vi "LED_test1.vi"() -> ()   [LabVIEW 2012]
uses:
  <vilib>/Utility/file.llb/Read From Spreadsheet File (DBL).vi
  <vilib>/gmath/NI_Gmath.lvlib
  <vilib>/Analysis/NI_AALPro.lvlib
panel:
  out "x2":dbl=3e-06
  out "x1":dbl=3e-06
  out "WL_1":dbl
  out "WL_2":dbl
  in  "WL2":dbl
  in  "WL1":dbl
  out "EQE_array":dbl[](array[numeric])
  out "XY Graph 4":T1(graph)
  out "XY Graph 3":cluster{"Wavelength":dbl[], "Counts":dbl[]}(graph)
  out "Luminance Ratio":dbl[](array[numeric])
  out "Calculated_luminance_array":dbl[](array[numeric])
  out "Calculated_candela_array":dbl[](array[numeric])
  out "Photon_count_array":dbl[](array[numeric])
  out "Photon_count":dbl
  out "Energy_WL":dbl[](array[numeric])
  out "Calculated_candela":dbl
  out "Abs_irr_itpl":dbl[](array[numeric]) format="%_6g"
  out "WL itpl 2":dbl[](array[numeric]) format="%_6g"
  out "Luminous Power Efficiency":dbl[](array[numeric])
  out "current efficiency (Cd/A)":dbl[](array[numeric])
  out "current density (mA/cm2)":dbl[](array[numeric])
  in  "Device Area (m2)":dbl=3e-06
  out "WL_spectrum":dbl[](array[numeric])
  out "Counts_spectrum":dbl[](array[numeric])
  out "Abs_Irr_spectrum":dbl[](array[numeric])
  out "subarray 2":dbl[][](array[numeric])
  out "Counts_dark_spectrum":dbl[](array[numeric])
  out "WL_dark_spectrum":dbl[](array[numeric])
  out "Dark Spectrum all":dbl[][](array[numeric]) format="%0.3f"
  out "Dark_spectrum":dbl[][](array[numeric])
  out "All Spectrum":dbl[][](array[numeric])
  in  "Spectrum File":path=path "W:/LED_quickVIEW/For calibration/20170914_194634spectrum_raw.ciemo"
  out "uW":dbl[](array[numeric])
  out "Luminance":dbl[](array[numeric])
  out "Candela":dbl[](array[numeric])
  out "Current":dbl[](array[numeric])
  out "Voltage":dbl[](array[numeric])
  out "Data":dbl[][](array[numeric]) format="%#.3e"
  out "Waveform Graph":T2(graph)
  in  "Data File":path=path "W:/LED_quickVIEW/For calibration/20170914_194634data.ciemo"
  in  "Calibration File":path=path "W:/LED_quickVIEW/For calibration/2016-12-19 callibration_OOIIrrad.cal_OOIIrrad.cal_OOIIrrad.cal"
  in  "Dark Spectrum File":path=path "W:/LED_quickVIEW/For calibration/20170914_194634dark_reference.ciemo"
  out "max value":dbl
  out "Peak Position":dbl
  out "max index(es)":i32
  out "Iso. Coef. itpl":dbl[](array[numeric]) format="%_6g"
  out "WL itpl":dbl[](array[numeric]) format="%_6g"
  out "XY Graph 2":cluster{"WL":dbl[], "Iso. Coef.":dbl[]}[](graph)
  out "Iso. Coef.":dbl[](array[numeric])
  out "WL":dbl[](array[numeric])
  out "Wavelength":dbl[](array[numeric])
  out "Counts to Abs Irr":dbl[](array[numeric])
  out "XY Graph":cluster{"Wavelength":dbl[], "Counts":dbl[]}(graph)
  out "subarray":dbl[][](array[numeric])
  out "array":dbl[][](array[numeric])
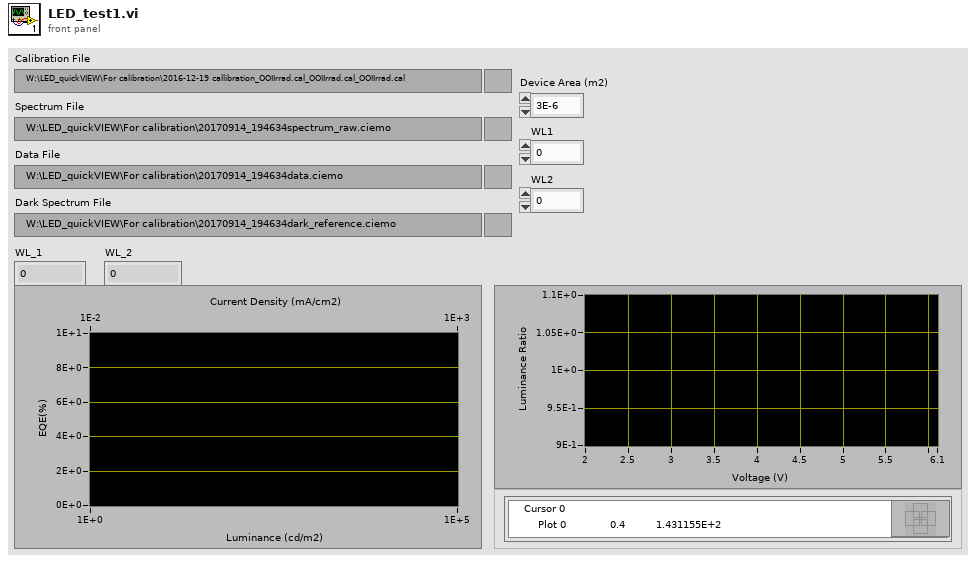
[diagram p1: front panel]
types:
  T1 = cluster{"current density (mA/cm2)":dbl[], "EQE_array":dbl[]}[]
  T2 = cluster{"min value":dbl, "min value":dbl, "Iso. Coef. itpl":dbl[]}
  T3 = cluster{"Wavelength":dbl[], "Counts to Abs Irr":dbl[]}
  T4 = cluster{"WL itpl":dbl[], "Iso. Coef. itpl":dbl[]}
  T5 = cluster{"WL itpl":dbl[], "Iso. Coef. itpl":dbl[]}[]
  T6 = cluster{"current density (mA/cm2)":dbl[], "EQE_array":dbl[]}
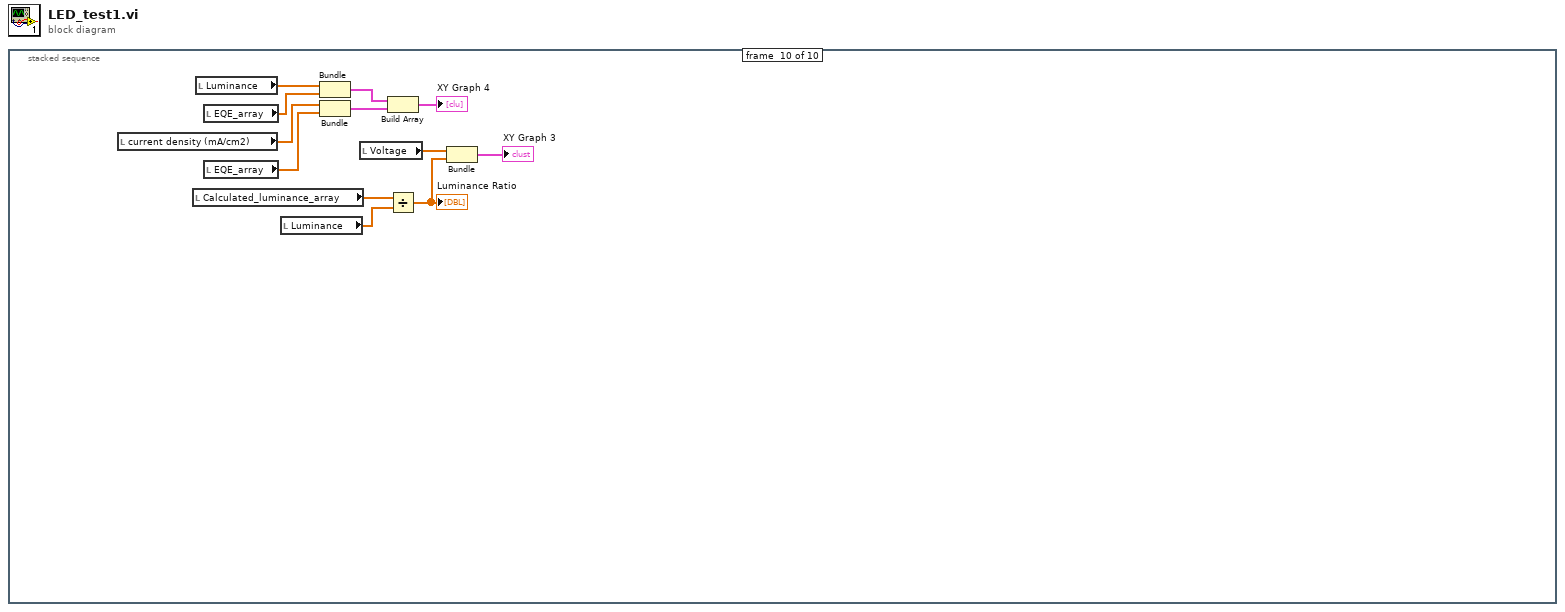
[diagram p0: block diagram]
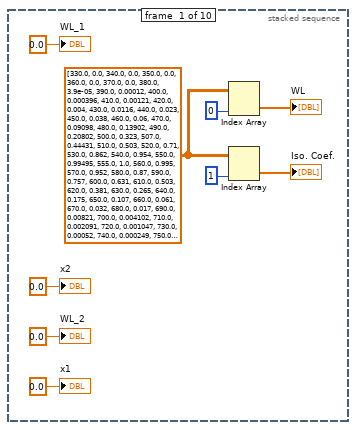
[diagram p2: hidden frame]
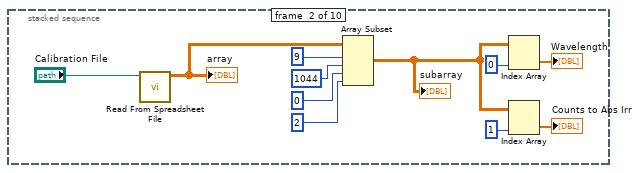
[diagram p3: hidden frame]
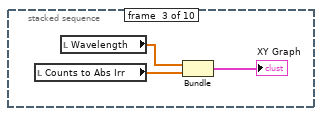
[diagram p4: hidden frame]
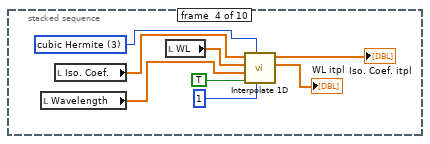
[diagram p5: hidden frame]
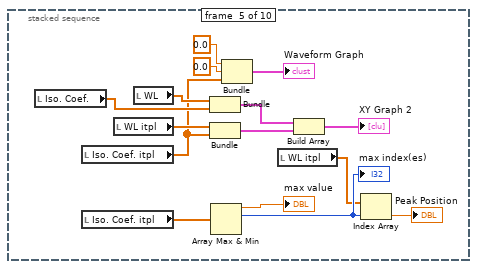
[diagram p6: hidden frame]
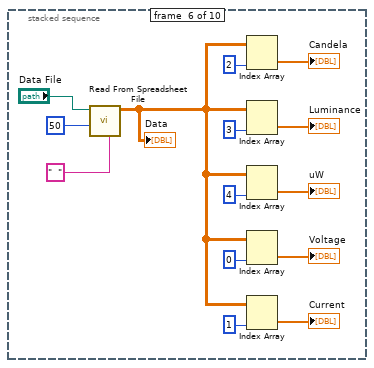
[diagram p7: hidden frame]
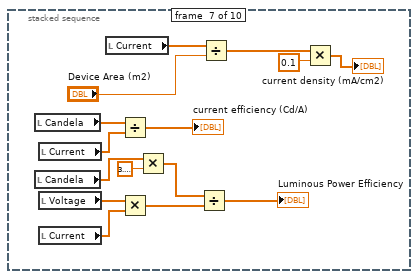
[diagram p8: hidden frame]
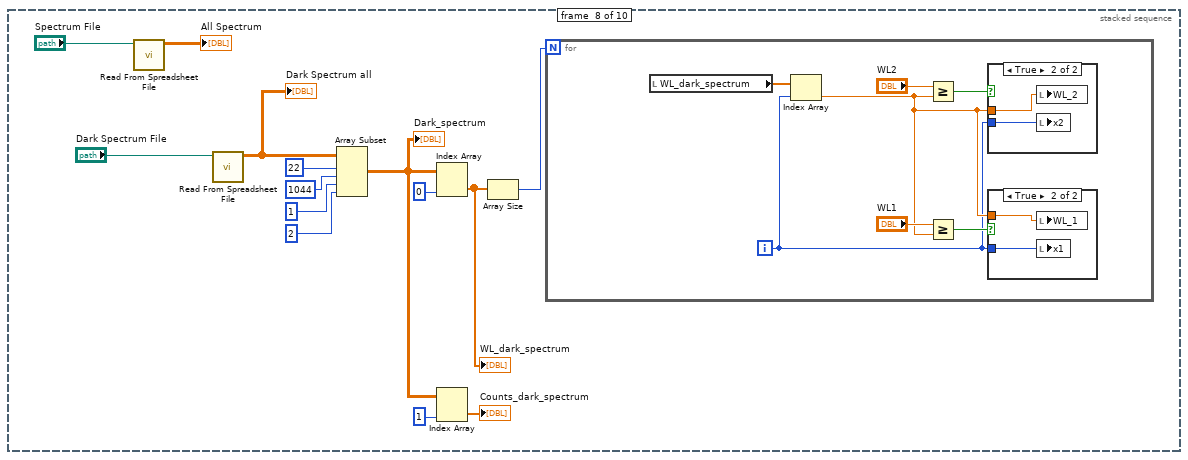
[diagram p9: hidden frame]
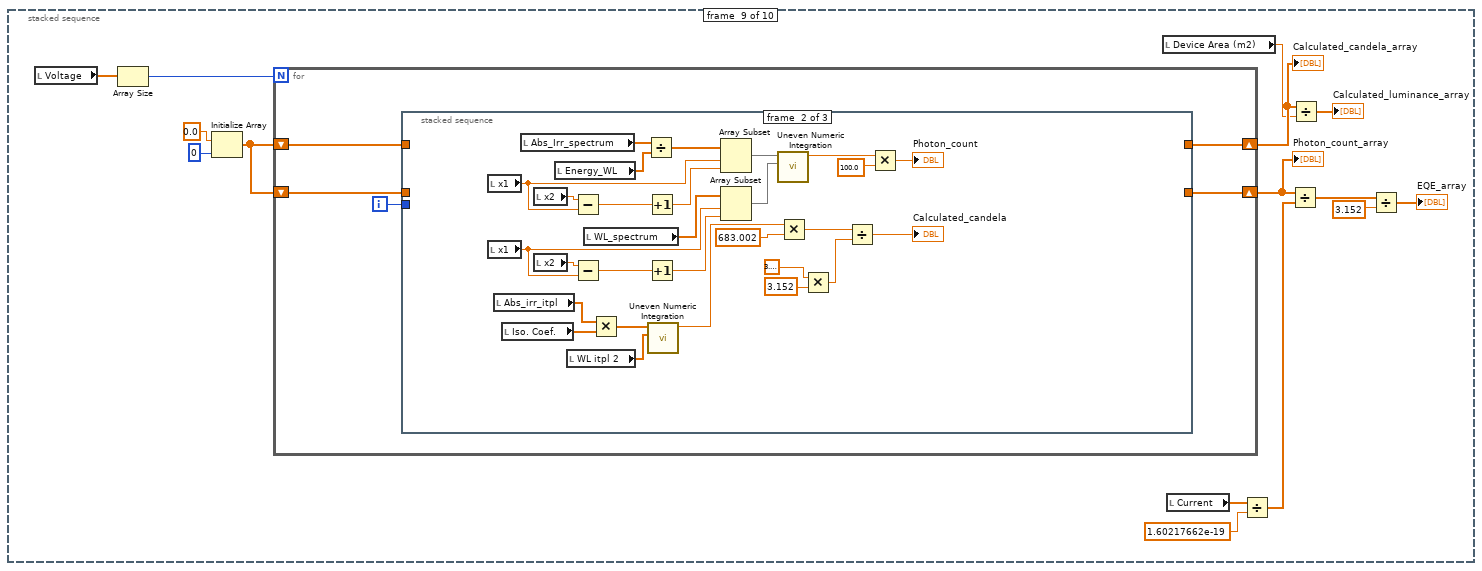
[diagram p12: hidden frame]
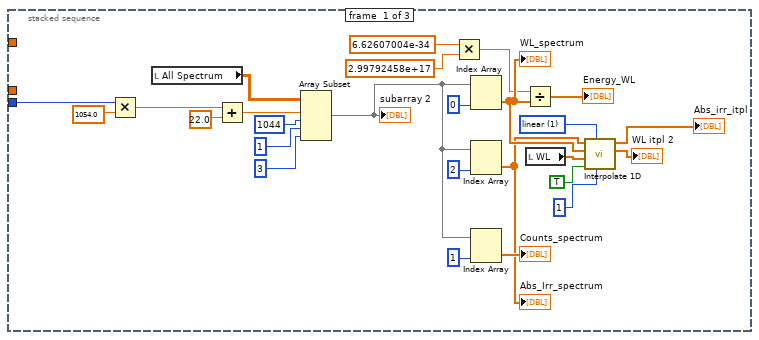
[diagram p13: hidden frame]
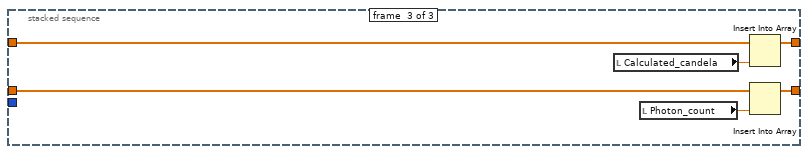
[diagram p14: hidden frame]
diagram:
  n1 = stacked-sequence {
    frame #0 {
      w8 = dbl[][] [[330.0, 0.0], [340.0, 0.0], [350.0, 0.0], [360.0, 0.0], [370.0, 0.0], [380.0, 3.9e-05], [390.0, 0.00012], [400.0, 0.000396], [410.0, 0.00121], [420.0, 0.004], [430.0, 0.0116], [440.0, 0.023], [450.0, 0.038], [460.0, 0.06], [470.0, 0.09098], [480.0, 0.13902], [490.0, 0.20802], [500.0, 0.323], [507.0, 0.44431], [510.0, 0.503], [520.0, 0.71], [530.0, 0.862], [540.0, 0.954], [550.0, 0.99495], [555.0, 1.0], [560.0, 0.995], [570.0, 0.952], [580.0, 0.87], [590.0, 0.757], [600.0, 0.631], [610.0, 0.503], [620.0, 0.381], [630.0, 0.265], [640.0, 0.175], [650.0, 0.107], [660.0, 0.061], [670.0, 0.032], [680.0, 0.017], [690.0, 0.00821], [700.0, 0.004102], [710.0, 0.002091], [720.0, 0.001047], [730.0, 0.00052], [740.0, 0.000249], [750.0, 0.00012], [760.0, 6e-05], [770.0, 3e-05], [780.0, 0.0], [790.0, 0.0], [800.0, 0.0], [810.0, 0.0], [820.0, 0.0], [830.0, 0.0], [840.0, 0.0], [850.0, 0.0], [860.0, 0.0], [870.0, 0.0], [880.0, 0.0], [890.0, 0.0], [900.0, 0.0], [910.0, 0.0], [920.0, 0.0], [930.0, 0.0], [940.0, 0.0], [950.0, 0.0], [960.0, 0.0], [970.0, 0.0], [980.0, 0.0], [990.0, 0.0], [1000.0, 0.0], [1010.0, 0.0], [1020.0, 0.0], [1030.0, 0.0], [1040.0, 0.0], [1050.0, 0.0], [1060.0, 0.0], [1070.0, 0.0], [1080.0, 0.0], [1090.0, 0.0], [1100.0, 0.0], [1110.0, 0.0], [1120.0, 0.0], [1130.0, 0.0], [1140.0, 0.0]] ("all rows")
      n2 = Index Array(array=w8, index (col)=0 ("disabled index (col)")) -> (element=→"WL":dbl[])  [unwired: 1 in]
      n3 = Index Array(array=w8, index (col)=1 ("disabled index (col)")) -> (element=→"Iso. Coef.":dbl[])  [unwired: 1 in]
      "WL_2" <- 0.0 ("WL_2")
      "WL_1" <- 0.0 ("WL_1")
      "x1" <- 0.0 ("x1")
      "x2" <- 0.0 ("x2")
    }
    frame #1 {
      n4 = call-poly <vilib>:"Read From Spreadsheet File.vi"("file path (dialog if empty)"="Calibration File") -> ("all rows"=w17:dbl[][])  [unwired: 6 in, 4 out]
      "array" <- w17
      n5 = Array Subset(array=w17, index (row)=9 ("index"), length (row)=1044 ("length"), index (col)=0 ("index"), length (col)=2 ("length")) -> (w14:dbl[][])
      "subarray" <- w14
      n6 = Index Array(array=w14, index (col)=0 ("index")) -> (element=→"Wavelength":dbl[])  [unwired: 1 in]
      n7 = Index Array(array=w14, index (col)=1 ("length")) -> (element=→"Counts to Abs Irr":dbl[])  [unwired: 1 in]
    }
    frame #2 {
      n8 = local read "Counts to Abs Irr"() -> (w21:dbl[])
      n9 = local read "Wavelength"() -> (w22:dbl[])
      n10 = Bundle("Wavelength"=w22, "Counts to Abs Irr"=w21) -> (→"XY Graph":T3)  [unwired: 1 in]
    }
    frame #3 {
      w27 = 3 items=["nearest", "linear", "spline", "cubic Hermite", "Lagrange"] ("method")
      n11 = local read "Wavelength"() -> (w29:dbl[])
      n12 = local read "Iso. Coef."() -> (w30:dbl[])
      n13 = local read "WL"() -> (w31:dbl[])
      n14 = call <vilib>:"Interpolate 1D.vi"("ntimes"=1, "method"=w27, "X is monotonic"=TRUE, "xi"=w29, "X"=w31, "Y"=w30) -> ("xi used"=→"WL itpl":dbl[], "yi"=→"Iso. Coef. itpl":dbl[])  [unwired: 3 in, 1 out]
    }
    frame #4 {
      n15 = local read "Iso. Coef."() -> (w46:dbl[])
      n16 = local read "Iso. Coef. itpl"() -> (w34:dbl[])
      n17 = local read "Iso. Coef. itpl"() -> (w39:dbl[])
      n18 = local read "WL itpl"() -> (w43:dbl[])
      n19 = local read "WL"() -> (w45:dbl[])
      n20 = Bundle("WL"=w45, "Iso. Coef."=w46) -> (w44:cluster{"WL":dbl[], "Iso. Coef.":dbl[]})  [unwired: 1 in]
      n21 = Bundle("WL itpl"=w43, "Iso. Coef. itpl"=w34) -> (w36:T4)  [unwired: 1 in]
      n22 = Array Max & Min(array=w39) -> (max value=→"max value":dbl, max index (indices)=w42:i32)  [unwired: 2 out]
      "max index(es)" <- w42
      n23 = Bundle("min value"=0.0, "min value"=0.0, "Iso. Coef. itpl"=w34) -> (→"Waveform Graph":T2)  [unwired: 1 in]
      n24 = local read "WL itpl"() -> (w41:dbl[])
      n25 = Build Array(w44, w36) -> (→"XY Graph 2":T5)
      n26 = Index Array(array=w41, index=w42) -> (element=→"Peak Position":dbl)
    }
    frame #5 {
      n27 = call-poly <vilib>:"Read From Spreadsheet File.vi"("delimiter (\\t)"="  " ("delimiter (\\t)"), "start of read offset (chars.:0)"=50, "file path (dialog if empty)"="Data File") -> ("all rows"=w47:dbl[][])  [unwired: 4 in, 4 out]
      "Data" <- w47
      n28 = Index Array(array=w47, index (col)=2 ("index (row)")) -> (element=→"Candela":dbl[])  [unwired: 1 in]
      n29 = Index Array(array=w47, index (col)=3 ("index (row)")) -> (element=→"Luminance":dbl[])  [unwired: 1 in]
      n30 = Index Array(array=w47, index (col)=4 ("index (row)")) -> (element=→"uW":dbl[])  [unwired: 1 in]
      n31 = Index Array(array=w47, index (col)=0 ("index (row)")) -> (element=→"Voltage":dbl[])  [unwired: 1 in]
      n32 = Index Array(array=w47, index (col)=1 ("index (row)")) -> (element=→"Current":dbl[])  [unwired: 1 in]
    }
    frame #6 {
      n33 = local read "Candela"() -> (w70:dbl[])
      n34 = local read "Candela"() -> (w63:dbl[])
      n35 = local read "Current"() -> (w71:dbl[])
      n36 = local read "Voltage"() -> (w65:dbl[])
      n37 = local read "Current"() -> (w64:dbl[])
      n38 = local read "Current"() -> (w68:dbl[])
      n39 = Divide(x=w70, y=w71) -> (x/y=→"current efficiency (Cd/A)":dbl[])
      n40 = Multiply(x=w65, y=w64) -> (x*y=w67:dbl[])
      n41 = Multiply(x=w63, y=3.141592653589793) -> (x*y=w66:dbl[])
      n42 = Divide(x=w66, y=w67) -> (x/y=→"Luminous Power Efficiency":dbl[])
      n43 = Divide(x=w68, y="Device Area (m2)") -> (x/y=w73:dbl[])
      n44 = Multiply(x=w73, y=0.1) -> (x*y=→"current density (mA/cm2)":dbl[])
    }
    frame #7 {
      n45 = call-poly <vilib>:"Read From Spreadsheet File.vi"("file path (dialog if empty)"="Spectrum File") -> ("all rows"=→"All Spectrum":dbl[][])  [unwired: 6 in, 4 out]
      n46 = call-poly <vilib>:"Read From Spreadsheet File.vi"("file path (dialog if empty)"="Dark Spectrum File") -> ("all rows"=w86:dbl[][])  [unwired: 6 in, 4 out]
      "Dark Spectrum all" <- w86
      n47 = Array Subset(array=w86, index (row)=22 ("index"), length (row)=1044 ("length"), index (col)=1 ("index"), length (col)=2 ("length")) -> (w78:dbl[][])
      "Dark_spectrum" <- w78
      n48 = Index Array(array=w78, index (col)=0 ("index")) -> (element=w77:dbl[])  [unwired: 1 in]
      "WL_dark_spectrum" <- w77
      n49 = Index Array(array=w78, index (col)=1 ("index")) -> (element=→"Counts_dark_spectrum":dbl[])  [unwired: 1 in]
      n50 = Array Size(array=w77) -> (size(s)=w76:i32)
      n51 = for {
        N: w76 -> [_]
        i -> [w90]
        n52 = local read "WL_dark_spectrum"() -> (w92:dbl[])
        n53 = Index Array(array=w92, index=w90) -> (element=w91:dbl)
        n54 = Greater Or Equal?(x="WL2", y=w91) -> (x >= y?=w94:bool)
        n55 = Greater Or Equal?(x="WL1", y=w91) -> (x >= y?=w93:bool)
        n56 = case shown="True" w94 {
          tunnel: w91 -> [_ w100]
          tunnel: w90 -> [_ w99]
          frame False {
          }
          frame True {
            n57 = local write "WL_2"(w100) -> ()
            n58 = local write "x2"(w99) -> ()
          }
        }
        n59 = case shown="True" w93 {
          tunnel: w91 -> [_ w98]
          tunnel: w90 -> [_ w97]
          frame False {
          }
          frame True {
            n60 = local write "WL_1"(w98) -> ()
            n61 = local write "x1"(w97) -> ()
          }
        }
      }
    }
    frame #8 {
      n62 = local read "Voltage"() -> (w115:dbl[])
      n63 = Array Size(array=w115) -> (size(s)=w114:i32)
      n64 = Initialize Array(0.0 ("element"), 0 ("dimension size")) -> (w111:dbl[])
      n65 = for {
        N: w114 -> [_]
        shift-right: [w118] -> w110
        shift-left: w111 -> [w119]
        shift-right: [w116] -> w105
        shift-left: w111 -> [w117]
        i -> [w120]
        n66 = stacked-sequence {
          tunnel: w120 -> [w134 _ _]
          tunnel: w119 -> [_ _ w179]
          tunnel: [_ _ w178] -> w118
          tunnel: w117 -> [_ _ w176]
          tunnel: [_ _ w175] -> w116
          frame #0 {
            w131 = 1 items=["nearest", "linear", "spline", "cubic Hermite", "Lagrange"] ("method")
            n67 = Multiply(x=w134, y=1054.0) -> (x*y=w144:dbl)
            n68 = local read "All Spectrum"() -> (w133:dbl[][])
            n69 = Add(x=w144, y=22.0) -> (x+y=w146:dbl)
            n70 = Array Subset(array=w133, index (row)=w146, length (row)=1044 ("length"), index (col)=1 ("index"), length (col)=3 ("length")) -> (w137:dbl[][])
            "subarray 2" <- w137
            n71 = Multiply(x=6.62607004e-34, y=2.99792458e+17) -> (x*y=w124:dbl)
            n72 = Index Array(array=w137, index (col)=0 ("index")) -> (element=w128:dbl[])  [unwired: 1 in]
            "WL_spectrum" <- w128
            n73 = Index Array(array=w137, index (col)=2 ("index")) -> (element=w127:dbl[])  [unwired: 1 in]
            "Abs_Irr_spectrum" <- w127
            n74 = Index Array(array=w137, index (col)=1 ("length")) -> (element=→"Counts_spectrum":dbl[])  [unwired: 1 in]
            n75 = Divide(x=w124, y=w128) -> (x/y=→"Energy_WL":dbl[])
            n76 = local read "WL"() -> (w126:dbl[])
            n77 = call <vilib>:"Interpolate 1D.vi"("ntimes"=1, "method"=w131, "X is monotonic"=TRUE, "xi"=w126, "X"=w128, "Y"=w127) -> ("xi used"=→"WL itpl 2":dbl[], "yi"=→"Abs_irr_itpl":dbl[])  [unwired: 3 in, 1 out]
          }
          frame #1 {
            n78 = local read "x1"() -> (w151:dbl)
            n79 = local read "x1"() -> (w149:dbl)
            n80 = local read "Abs_irr_itpl"() -> (w174:dbl[])
            n81 = local read "Iso. Coef."() -> (w173:dbl[])
            n82 = local read "Abs_Irr_spectrum"() -> (w166:dbl[])
            n83 = local read "x2"() -> (w152:dbl)
            n84 = local read "x2"() -> (w150:dbl)
            n85 = local read "Energy_WL"() -> (w165:dbl[])
            n86 = local read "WL itpl 2"() -> (w171:dbl[])
            n87 = Subtract(x=w152, y=w151) -> (x-y=w157:dbl)
            n88 = Subtract(x=w150, y=w149) -> (x-y=w154:dbl)
            n89 = local read "WL_spectrum"() -> (w148:dbl[])
            n90 = Multiply(x=w174, y=w173) -> (x*y=w172:dbl[])
            n91 = Divide(x=w166, y=w165) -> (x/y=w158:dbl[])
            n92 = Increment(x=w157) -> (x+1=w156:dbl)
            n93 = Increment(x=w154) -> (x+1=w153:dbl)
            n94 = call <vilib>:"Uneven Numeric Integration.vi"("T"=w171, "X"=w172) -> ("result"=w169:dbl)  [unwired: 8 in, 1 out]
            n95 = Array Subset(array=w158, index=w151, length=w156) -> (w155:dbl[])
            n96 = Array Subset(array=w148, index=w149, length=w153) -> (w147:dbl[])
            n97 = call <vilib>:"Uneven Numeric Integration.vi"("T"=w147, "X"=w155) -> ("result"=w164:dbl)  [unwired: 8 in, 1 out]
            n98 = Multiply(x=w169, y=683.002) -> (x*y=w170:dbl)
            n99 = Multiply(x=3.141592653589793, y=3.152) -> (x*y=w160:dbl)
            n100 = Divide(x=w170, y=w160) -> (x/y=→"Calculated_candela":dbl)
            n101 = Multiply(x=w164, y=100.0) -> (x*y=→"Photon_count":dbl)
          }
          frame #2 {
            n102 = local read "Calculated_candela"() -> (w180:dbl)
            n103 = local read "Photon_count"() -> (w177:dbl)
            n104 = Insert Into Array(array=w179, new element=w180) -> (w178:dbl[])  [unwired: 1 in]
            n105 = Insert Into Array(array=w176, new element=w177) -> (w175:dbl[])  [unwired: 1 in]
          }
        }
      }
      "Photon_count_array" <- w105
      "Calculated_candela_array" <- w110
      n106 = local read "Device Area (m2)"() -> (w108:dbl)
      n107 = local read "Current"() -> (w107:dbl[])
      n108 = Divide(x=w107, y=1.60217662e-19) -> (x/y=w106:dbl[])
      n109 = Divide(x=w105, y=w106) -> (x/y=w103:dbl[])
      n110 = Divide(x=w110, y=w108) -> (x/y=→"Calculated_luminance_array":dbl[])
      n111 = Divide(x=w103, y=3.152) -> (x/y=→"EQE_array":dbl[])
    }
    frame #9 {
      n112 = local read "current density (mA/cm2)"() -> (w184:dbl[])
      n113 = local read "Calculated_luminance_array"() -> (w191:dbl[])
      n114 = local read "Luminance"() -> (w185:dbl[])
      n115 = local read "EQE_array"() -> (w186:dbl[])
      n116 = local read "EQE_array"() -> (w187:dbl[])
      n117 = local read "Luminance"() -> (w192:dbl[])
      n118 = Bundle("Luminance"=w185, "EQE_array"=w186) -> (w183:cluster{"Luminance":dbl[], "EQE_array":dbl[]})  [unwired: 1 in]
      n119 = Bundle("current density (mA/cm2)"=w184, "EQE_array"=w187) -> (w182:T6)  [unwired: 1 in]
      n120 = local read "Voltage"() -> (w190:dbl[])
      n121 = Build Array(w183, w182) -> (→"XY Graph 4":T1)
      n122 = Divide(x=w191, y=w192) -> (x/y=w189:dbl[])
      "Luminance Ratio" <- w189
      n123 = Bundle("Voltage"=w190, w189) -> (→"XY Graph 3":cluster{"Voltage":dbl[], dbl[]})  [unwired: 1 in]
    }
  }
